vi "Newport ITX-D3N Zero Filter.vi"(6 "element 5":dbl, 8 "element 4":dbl, 9 "element 3":dbl, 10 "element 2":dbl, 11 "element":dbl) -> (3 "median":dbl format="%0.2f")   [LabVIEW 2018]
uses:
  <vilib>/Analysis/NI_AALBase.lvlib
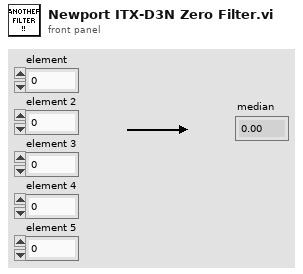
[diagram p1: front panel]
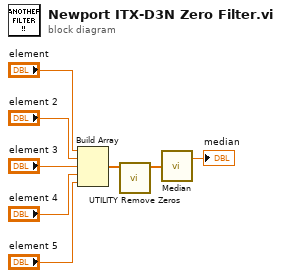
[diagram p0: block diagram]
diagram:
  n1 = Build Array("element", "element 2", "element 3", "element 4", "element 5") -> (w3:dbl[])
  n2 = call "UTILITY Remove Zeros.vi"("Array in"=w3) -> ("Array out"=w2:dbl[])  [unwired: 10 in]
  n3 = call <vilib>:"Median.vi"("X"=w2) -> ("median"=→"median":dbl)  [unwired: 1 out]
